vi "Build Filter.vi"(6 "Filter Type":T1, 7 "Time Filter Configuration":T5, 8 "error in (no error)":errorcluster, 9 "Boolean Filter Configuration":T2, 10 "String Filter Configuration":T3) -> (0 "error out":errorcluster, 2 "Base Filter out":refnum<class "Base Filter.lvclass">, 5 "Boolean":bool)   [LabVIEW 2016, in "Assert API Components.lvlib" / "Assert Display.lvlib"]
uses:
  Assert Display.lvlib
  Assert API Components/Time Filter Configuration.ctl
  Assert API Components/Filter By Time.ctl
  Assert API Components/String Filter Configuration.ctl
  Assert API Components/Filter By String.ctl
  Assert API Components/Boolean Filter Configuration.ctl
  Assert API Components/Filter Type.ctl
  Assert API Components/Filter Configurations/Base Filter.lvclass
  Assert API Components/Filter Configurations/Status Filter/Status.lvclass
  C:/Users/ukhornp/Documents/Work/Projects/actor_assert_api/Core/Assert API Components/Filter Configurations/Base Filter.lvclass
  C:/Users/ukhornp/Documents/Work/Projects/actor_assert_api/Core/Assert API Components/Filter Configurations/Boolean Filters/Boolean Filter.lvclass
  Assert API Components/Filter Configurations/Assert Builder User Name Filter/Assert Builder User Name.lvclass
  C:/Users/ukhornp/Documents/Work/Projects/actor_assert_api/Core/Assert API Components/Filter Configurations/String Filters/String Filters.lvclass
  Assert API Components/Filter Configurations/Assert Name Filter/Assert Name Filter.lvclass
  Assert API Components/Filter Configurations/Assert VI Name Filter/Assert VI Name.lvclass
  Assert API Components/Filter Configurations/Calling VI Name Filter/Calling VI Name.lvclass
  Assert API Components/Filter Configurations/Comment Filter/Comment.lvclass
  Assert API Components/Filter Configurations/Data Type Filter/Data Type.lvclass
  Assert API Components/Filter Configurations/Evaluation String Filter/Evaluation String.lvclass
  Assert API Components/Filter Configurations/Assert Build Timestamp Filter/Assert Build Timestamp Filter.lvclass
  C:/Users/ukhornp/Documents/Work/Projects/actor_assert_api/Core/Assert API Components/Filter Configurations/Time Filters/Time Filters.lvclass
  Assert API Components/Filter Configurations/Last Update Timestamp Filter/Last Update Timestamp Filter.lvclass
  Assert API Components/Filter Configurations/String Filters/String Filters.lvclass
  Assert API Components/Filter Configurations/Time Filters/Time Filters.lvclass
  Assert API Components/Filter Configurations/Boolean Filters/Boolean Filter.lvclass
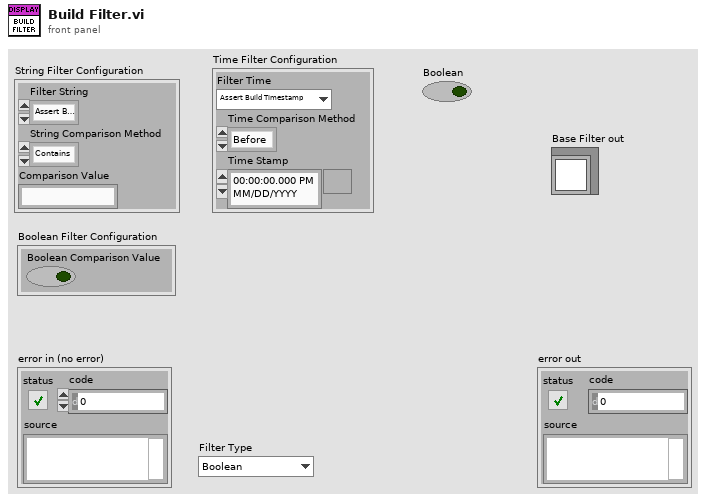
[diagram p1: front panel]
types:
  T1 = typedef "Assert API Components.lvlib/Assert Display.lvlib/Filter Type.ctl" = enum16{"Boolean", "String", "Time"}
  T2 = typedef "Assert API Components.lvlib/Assert Display.lvlib/Boolean Filter Configuration.ctl" = cluster{"Boolean Comparison Value":bool}
  T3 = typedef "Assert API Components.lvlib/Assert Display.lvlib/String Filter Configuration.ctl" = cluster{"Filter String":T4, "String Comparison Method":enum16{"Contains", "Does Not Contain", "Starts With", "Equals", "Does Not Equal"}, "Comparison Value":string}
  T4 = typedef "Assert API Components.lvlib/Assert Display.lvlib/Filter By String.ctl" = enum16{"Assert Builder User Name", "Assert Name", "Assert VI Name", "Calling VI Name", "Comment", "Data Type", "Evaluation String"}
  T5 = typedef "Assert API Components.lvlib/Assert Display.lvlib/Time Filter Configuration.ctl" = cluster{"Filter Time":T6, "Time Comparison Method":enum16{"Before", "After"}, "Time Stamp":timestamp}
  T6 = typedef "Assert API Components.lvlib/Assert Display.lvlib/Filter By Time.ctl" = enum16{"Assert Build Timestamp", "Last Update Timestamp"}
  T7 = enum16{"Contains", "Does Not Contain", "Starts With", "Equals", "Does Not Equal"}
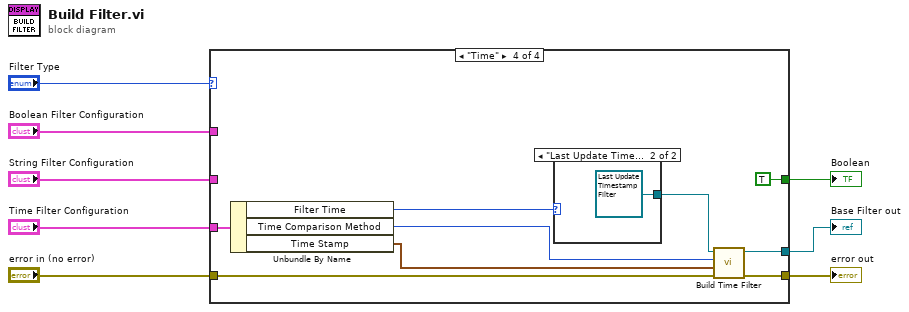
[diagram p0: block diagram]
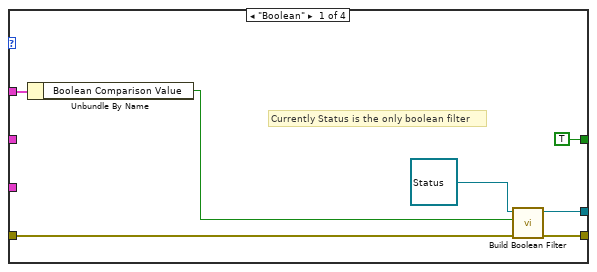
[diagram p2: hidden frame]
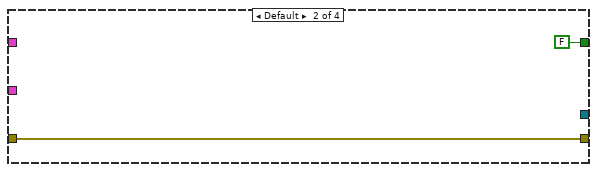
[diagram p3: hidden frame]
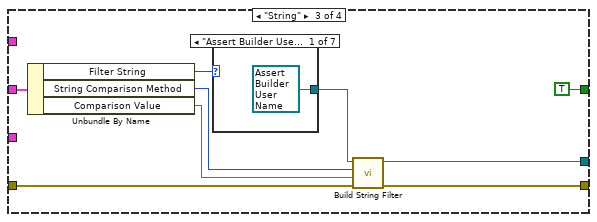
[diagram p4: hidden frame]
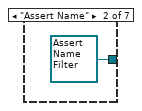
[diagram p5: hidden frame]
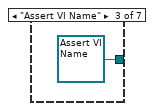
[diagram p6: hidden frame]
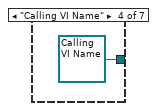
[diagram p7: hidden frame]
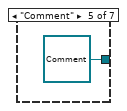
[diagram p8: hidden frame]
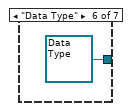
[diagram p9: hidden frame]
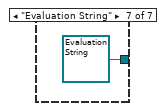
[diagram p10: hidden frame]
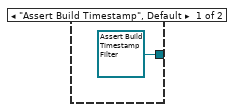
[diagram p11: hidden frame]
diagram:
  n1 = case shown="\"Time\"" "Filter Type" {
    tunnel: [w12 w16 w26 w40] -> w1
    tunnel: [w13 _ w25 w41] -> w2
    tunnel: [TRUE FALSE TRUE TRUE] -> w4
    tunnel: "Boolean Filter Configuration" -> [w11 _ _ _]
    tunnel: "String Filter Configuration" -> [_ _ w21 _]
    tunnel: "Time Filter Configuration" -> [_ _ _ w38]
    tunnel: "error in (no error)" -> [w9 w16 w22 w34]
    frame "Boolean" {
      # "Currently Status is the only boolean filter"
      n2 = Unbundle By Name(w11) -> ("Boolean Comparison Value"=w10:bool)
      n3 = call "Build Boolean Filter.vi"("error in (no error)"=w9, "Comparision Value"=w10, "Boolean Filter in"=refnum<class "Status.lvclass"> refnum ("Assert API Components.lvlib:Status.lvclass")) -> ("error out"=w12:errorcluster, "Boolean Filter out"=w13:refnum<class "Status.lvclass">)  [unwired: 7 in]
    }
    frame Default {
    }
    frame "String" {
      n4 = Unbundle By Name(w21) -> ("Filter String"=w18:T4, "String Comparison Method"=w20:T7, "Comparison Value"=w19:string)
      n5 = case shown="\"Assert Builder User Name\", Default" w18 {
        tunnel: [refnum<class "Assert Builder User Name.lvclass"> refnum ("Assert API Components.lvlib:Assert Builder User Name.lvclass") refnum<class "Assert Name Filter.lvclass"> refnum ("Assert API Components.lvlib:Assert Name Filter.lvclass") refnum<class "Assert VI Name.lvclass"> refnum ("Assert API Components.lvlib:Assert VI Name.lvclass") refnum<class "Calling VI Name.lvclass"> refnum ("Assert API Components.lvlib:Calling VI Name.lvclass") refnum<class "Comment.lvclass"> refnum ("Assert API Components.lvlib:Comment.lvclass") refnum<class "Data Type.lvclass"> refnum ("Assert API Components.lvlib:Data Type.lvclass") refnum<class "Evaluation String.lvclass"> refnum ("Assert API Components.lvlib:Evaluation String.lvclass")] -> w24
        frame "Assert Builder User Name", Default {
        }
        frame "Assert Name" {
        }
        frame "Assert VI Name" {
        }
        frame "Calling VI Name" {
        }
        frame "Comment" {
        }
        frame "Data Type" {
        }
        frame "Evaluation String" {
        }
      }
      n6 = call-dynamic "Build String Filter.vi"("error in (no error)"=w22, "Comparison Value"=w19, "Comparison Method"=w20, "String Filters in"=w24) -> ("error out"=w26:errorcluster, "String Filters out"=w25:refnum<class "String Filters.lvclass">)  [unwired: 6 in]
    }
    frame "Time" {
      n7 = Unbundle By Name(w38) -> ("Filter Time"=w37:T6, "Time Comparison Method"=w36:enum16{"Before", "After"}, "Time Stamp"=w35:timestamp)
      n8 = case shown="\"Last Update Timestamp\"" w37 {
        tunnel: [refnum<class "Assert Build Timestamp Filter.lvclass"> refnum ("Assert API Components.lvlib:Assert Build Timestamp Filter.lvclass") refnum<class "Last Update Timestamp Filter.lvclass"> refnum ("Assert API Components.lvlib:Last Update Timestamp Filter.lvclass")] -> w42
        frame "Assert Build Timestamp", Default {
        }
        frame "Last Update Timestamp" {
        }
      }
      n9 = call "Build Time Filter.vi"("error in (no error)"=w34, "Comparison Timestamp"=w35, "Comparison Method"=w36, "Time Filters in"=w42) -> ("error out"=w40:errorcluster, "Time Filters out"=w41:refnum<class "Time Filters.lvclass">)  [unwired: 6 in]
    }
  }
  "Boolean" <- w4
  "Base Filter out" <- w2
  "error out" <- w1
